vi "TCP_email_comms.vi"(0 "Commands Array":string[](array[string])) -> (1 "Replys":string[](array[string]), 2 "error out":errorcluster)   [LabVIEW 2010]
uses:
  Globals/Preference_global.vi
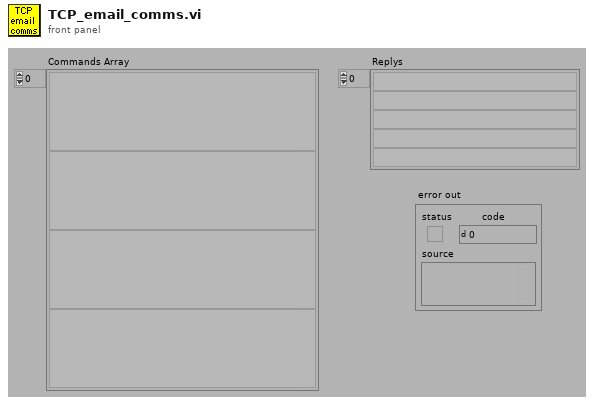
[diagram p1: front panel]
types:
  T1 = enum16{"Standard", "Buffered", "CRLF", "Immediate"}
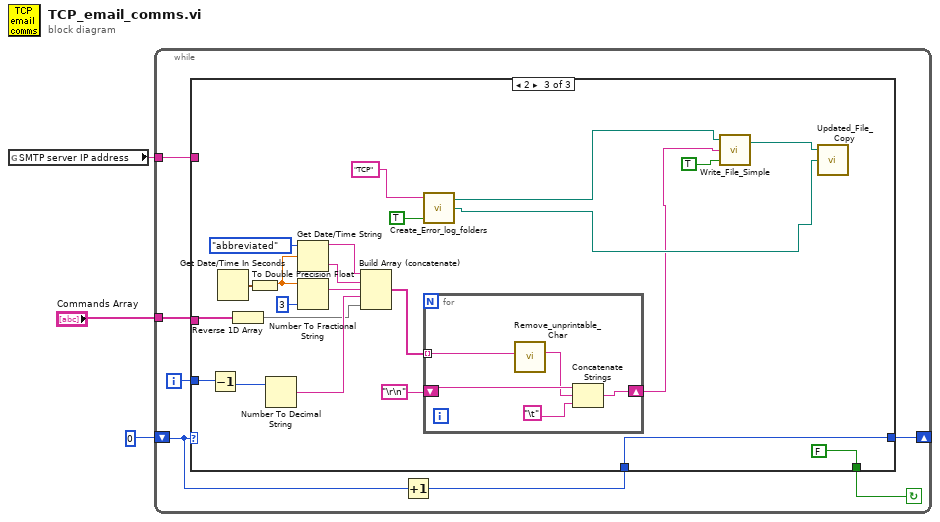
[diagram p0: block diagram]
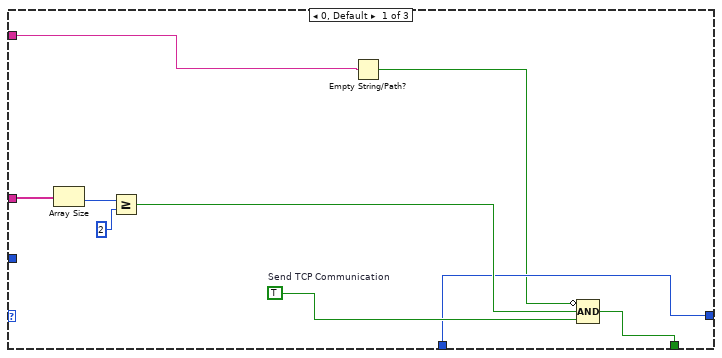
[diagram p2: hidden frame]
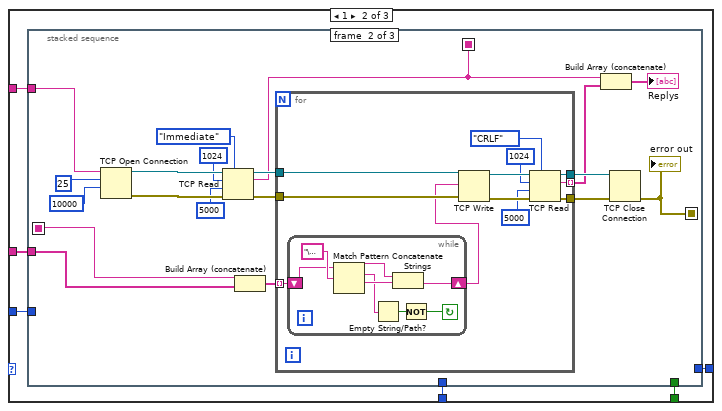
[diagram p3: hidden frame]
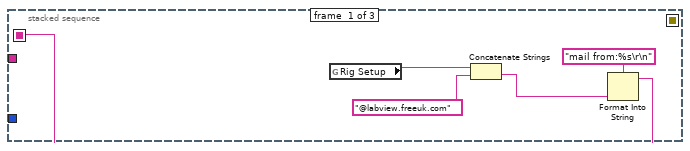
[diagram p4: hidden frame]
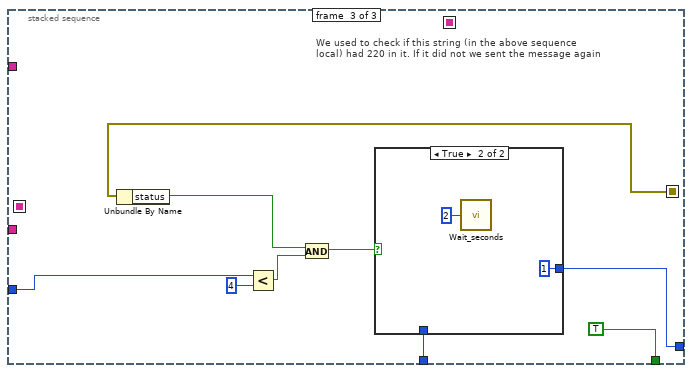
[diagram p5: hidden frame]
diagram:
  n1 = global read "Preference_global.vi" "SMTP server IP address"() -> (w1:string)
  n2 = while {
    tunnel: w1 -> [w4]
    shift-left: 0 -> [w8]
    shift-right: [w7] -> _
    tunnel: "Commands Array" -> [w10]
    i -> [w5]
    stop <- w9 continue-if-true
    n3 = Increment(x=w8) -> (x+1=w6:i32)
    n4 = case shown="2" w8 {
      tunnel: w10 -> [w17 w25 w100]
      tunnel: [w14 w24 FALSE] -> w9
      tunnel: [w13 w22 w98] -> w7
      tunnel: w6 -> [w13 w21 w98]
      tunnel: w5 -> [_ w23 w97]
      tunnel: w4 -> [w12 w20 _]
      frame 0, Default {
        w16 = TRUE  # Send TCP Communication
        n5 = Array Size(array=w17) -> (size(s)=w18:i32)
        n6 = Greater Or Equal?(x=w18, y=2) -> (x >= y?=w15:bool)
        n7 = Empty String/Path?(string/path=w12) -> (empty?=w11:bool)
        n8 = Compound Arithmetic op=AND(invert w11, w15, w16) -> (w14:bool)
      }
      frame 1 {
        n9 = stacked-sequence {
          seq-local: [w29 _ _] -> [_ w36 _]
          seq-local: [_ w34 _] -> [_ _ _]
          seq-local: [_ w33 _] -> [_ _ w78]
          tunnel: w25 -> [_ w38 _]
          tunnel: [_ _ TRUE] -> w24
          tunnel: w23 -> [_ _ w76]
          tunnel: [_ _ w72] -> w22
          tunnel: w21 -> [_ _ w71]
          tunnel: w20 -> [_ w31 _]
          frame #0 {
            n10 = global read "Preference_global.vi" "Rig Setup"() -> (w26:string)
            n11 = Concatenate Strings(w26, "@labview.freeuk.com" ("Mail from")) -> (w27:string)
            n12 = Format Into String(format string="mail from:%s\r\n" ("Format String"), w27) -> (resulting string=w29:string)  [unwired: 2 in, 1 out]
          }
          frame #1 {
            n13 = TCP Open Connection(address=w31, remote port or service name=u16 25, timeout ms (60000)=10000) -> (connection ID=w45:refnum<k5>, error out=w46:errorcluster)  [unwired: 1 in, 1 out]
            n14 = TCP Read(connection ID=w45, bytes to read=1024, error in (no error)=w46, 7:T1."Immediate" ("mode (standard)"), 9:5000 ("timeout ms (25000)")) -> (connection ID out=w47:refnum<k5>, data out=w34:string, error out=w49:errorcluster)
            n15 = Build Array (concatenate)(w36, w38) -> (w37:string[])
            n16 = for {
              tunnel: w47 -> [w61]
              tunnel: w49 -> [w60]
              tunnel: [w58] -> w48
              tunnel: [w54] -> w39 mode=indexing
              tunnel: [w52] -> w40
              tunnel: w37 -> [w51] mode=indexing
              n17 = while {
                shift-left: w51 -> [w68]
                shift-right: [w65] -> w50
                stop <- w62 continue-if-true
                n18 = Match Pattern(string=w68, regular expression="\u0000") -> (before substring=w67:string, match substring=w64:string, after substring=w66:string)  [unwired: 2 out]
                n19 = Empty String/Path?(string/path=w64) -> (empty?=w63:bool)
                n20 = Concatenate Strings(w67, w66) -> (w65:string)
                n21 = Not(x=w63) -> (.not. x?=w62:bool)
              }
              n22 = TCP Write(connection ID=w61, data in=w50, error in (no error)=w60) -> (connection ID out=w59:refnum<k5>, error out=w57:errorcluster)  [unwired: 2 out]
              n23 = TCP Read(connection ID=w59, bytes to read=1024, error in (no error)=w57, 7:T1."CRLF" ("mode (standard)"), 9:5000 ("timeout ms (25000)")) -> (connection ID out=w58:refnum<k5>, data out=w54:string, error out=w52:errorcluster)
            }
            n24 = Build Array (concatenate)(w34, w39) -> (→"Replys":string[])
            n25 = TCP Close Connection(connection ID=w48, error in (no error)=w40) -> (error out=w33:errorcluster)  [unwired: 1 in, 1 out]
            "error out" <- w33
          }
          frame #2 {
            # "We used to check if this string (in the above sequence local) had 220 in it. If it did not we sent the message again"
            n26 = Unbundle By Name(w78) -> ("status"=w70:bool)
            n27 = Less?(x=w76, y=4) -> (x < y?=w74:bool)
            n28 = And(x=w70, y=w74) -> (x .and. y?=w73:bool)
            n29 = case shown="True" w73 {
              tunnel: [w79 1] -> w72
              tunnel: w71 -> [w79 _]
              frame False {
              }
              frame True {
                n30 = call "Wait_seconds.vi"("Seconds to wait"=u32 2) -> ()
              }
            }
          }
        }
      }
      frame 2 {
        n31 = Decrement(x=w97) -> (x-1=w96:i32)
        n32 = Get Date/Time In Seconds() -> (seconds since 1Jan1904=w88:timestamp)
        n33 = Reverse 1D Array(array=w100) -> (reversed array=w93:string[])
        n34 = To Double Precision Float(number=w88) -> (double precision float=w90:dbl)
        n35 = Number To Decimal String(number=w96) -> (decimal integer string=w95:string)  [unwired: 1 out]
        n36 = Get Date/Time String(date format (0)=enum16{"short", "long", "abbreviated"}."abbreviated", seconds (now)=w90) -> (date string=w104:string, time string=w103:string)  [unwired: 1 out]
        n37 = Number To Fractional String(number=w90, precision (6)=i16 3) -> (F-format string=w89:string)  [unwired: 2 out]
        n38 = Build Array (concatenate)(w104, w103, w89, w95, w93) -> (w102:string[])
        n39 = call "Create_Error_log_folders.vi"("Per Day Log File?"=TRUE, "Log Filename"="TCP" ("Input Element")) -> ("Server copy Location"=w87:path, "Local Log File"=w86:path)  [unwired: 1 in, 1 out]
        n40 = for {
          tunnel: w102 -> [w109] mode=indexing
          shift-right: [w106] -> w85
          shift-left: "\r\n" -> [w108]
          n41 = call "Remove_unprintable_Char.vi"("Input String"=w109) -> ("Output String"=w107:string)
          n42 = Concatenate Strings(w108, w107, "\t") -> (w106:string)
        }
        n43 = call "Write_File_Simple.vi"("append to file? (new file:F)"=TRUE, "character string"=w85, "file path"=w86) -> ("file path Out"=w83:path)  [unwired: 1 out]
        n44 = call "Updated_File_Copy.vi"("Target Path"=w87, "Source Path"=w83) -> ()  [unwired: 2 out]
      }
    }
  }
